vi "Joystick To Discreet Angles.vi"(8 "Deadband":dbl=0.85, 9 "Zones":i32, 10 "Y":dbl(slide) scale=1.0..-1.0, 11 "X":dbl(slide) scale=-1.0..1.0) -> (1 "Valid":bool, 2 "Discreet Angle":i32, 3 "Angle":dbl)   [LabVIEW 2019]
panel:
  # "315"
  # "0"
  # "45"
  # "Joystick"
  # "270"
  # "90"
  # "225"
  # "180"
  # "135"
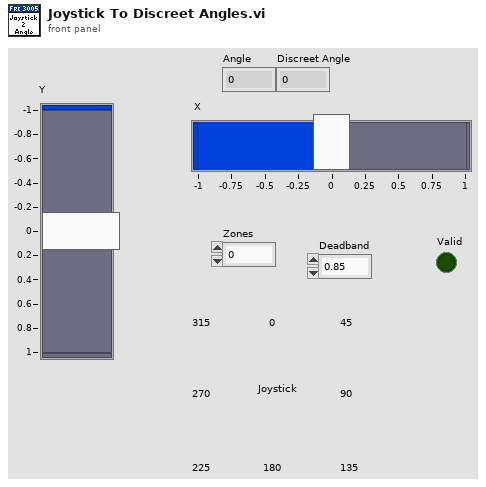
[diagram p1: front panel]
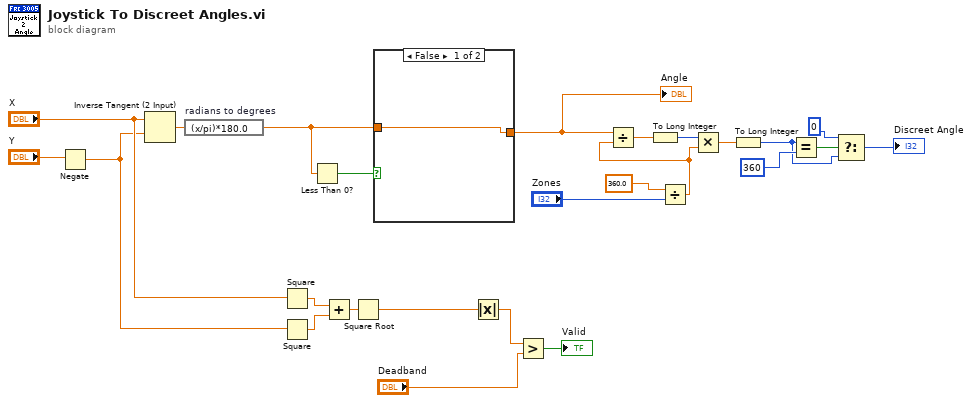
[diagram p0: block diagram]
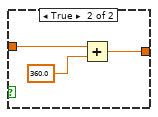
[diagram p2: hidden frame]
diagram:
  n1 = Negate(x="Y") -> (-x=w7:dbl)
  n2 = Inverse Tangent (2 Input)(1:w7, 2:"X") -> (0:w25:dbl)
  n3 = expression code="(x/pi)*180.0" "radians to degrees"(w25) -> (w22:dbl)
  n4 = Square(x="X") -> (x^2=w13:dbl)
  n5 = Square(x=w7) -> (x^2=w12:dbl)
  n6 = Less Than 0?(x=w22) -> (x < 0?=w23:bool)
  n7 = Add(x=w13, y=w12) -> (x+y=w11:dbl)
  n8 = Square Root(x=w11) -> (sqrt(x)=w10:dbl)
  n9 = case shown="False" w23 {
    tunnel: w22 -> [w26 w29]
    tunnel: [w26 w27] -> w21
    frame False {
    }
    frame True {
      n10 = Add(x=w29, y=360.0) -> (x+y=w27:dbl)
    }
  }
  "Angle" <- w21
  n11 = Absolute Value(x=w10) -> (abs(x)=w14:dbl)
  n12 = Greater?(x=w14, y="Deadband") -> (0:→"Valid":bool)
  n13 = Divide(x=360.0, y="Zones") -> (x/y=w16:dbl)
  n14 = Divide(x=w21, y=w16) -> (x/y=w18:dbl)
  n15 = To Long Integer(number=w18) -> (32bit integer=w17:i32)
  n16 = Multiply(x=w17, y=w16) -> (x*y=w15:dbl)
  n17 = To Long Integer(number=w15) -> (32bit integer=w3:i32)
  n18 = Equal?(x=w3, y=360) -> (x = y?=w4:bool)
  n19 = Select(t=0, s=w4, f=w3) -> (s? t:f=→"Discreet Angle":i32)
